vi "Demo.vi"() -> ()   [LabVIEW 2021, in "VI-Hacker.lvlib"]
uses:
  VI-Hacker.lvlib
panel:
  out "error out":errorcluster
  in  "Password Protected VI Path":path
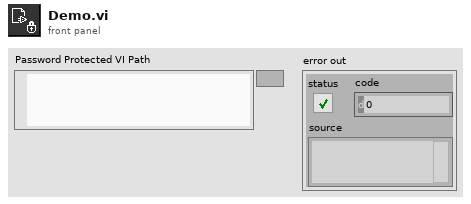
[diagram p1: front panel]
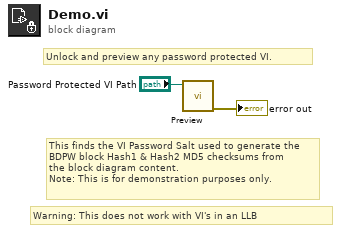
[diagram p0: block diagram]
diagram:
  # "Warning: This does not work with VI's in an LLB"
  # "This finds the VI Password Salt used to generate the\nBDPW block Hash1 & Hash2 MD5 checksums from\nthe block diagram content.\nNote: This is for demonstration purposes only."
  # "Unlock and preview any password protected VI."
  n1 = call "Preview.vi"("Password Protected VI Path"="Password Protected VI Path") -> ("error out"=→"error out":errorcluster)  [unwired: 10 in]
